vi "CL-close-CAN-test.vi"() -> ()   [LabVIEW 2016]
uses:
  <vilib>/Platform/TimedLoop/XDataNode/timing_clust.ctl
  <vilib>/Platform/TimedLoop/XDataNode/nitl_modes.ctl
  <vilib>/Platform/TimedLoop/XDataNode/wakeup.ctl
  <vilib>/xnet/xnet.llb/XNET Write (Signal Single-point).vi
  <vilib>/Platform/TimedLoop/XDataNode/XDataNode.xnode
  <vilib>/Platform/TimedLoop/XDataNode/XDNodeRunTimeDep.lvlib
panel:
  in  "Period":i64=10
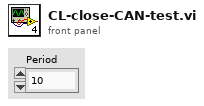
[diagram p1: front panel]
types:
  T1 = typedef "XDNodeRunTimeDep.lvlib/timing_clust.ctl" = cluster{"Expected End [f-1]":u64, "Actual End [f-1]":u64, "Finished Late? [f-1]":bool, "Expected End [i-1]":u64, "Actual End [i-1]":u64, "Finished Late? [i-1]":bool, "Expected Start [i]":u64, "Actual Start [i]":u64, "Expected Start [f]":u64, "Actual Start [f]":u64, "Source Name":string, "Structure Name":string, "Period":i64, "Deadline":i64, "Offset":i64, "Start":i64, "Priority":i32, "Timeout":i32, "Mode":T2, "Wakeup Reason":T3, "Error":errorcluster, "Source Type":string, "Secondary Source Type":string, "Global End Time":u64, "Global Start Time":u64, "Frame Duration":u64, "Iteration Duration":u64, "Assigned CPU":i32, "I/O Scan Engine Mode":u32}
  T2 = typedef "XDNodeRunTimeDep.lvlib/nitl_modes.ctl" = enum32{"No Change", "Process missed periods, maintain original phase", "Discard missed periods, maintain original phase", "Process missed periods, ignore original phase", "Discard missed periods, ignore original phase"}
  T3 = typedef "XDNodeRunTimeDep.lvlib/wakeup.ctl" = enum32{"Normal", "Aborted", "Asynchronous wakeup", "Timing source error", "Timed loop error", "Timeout"}
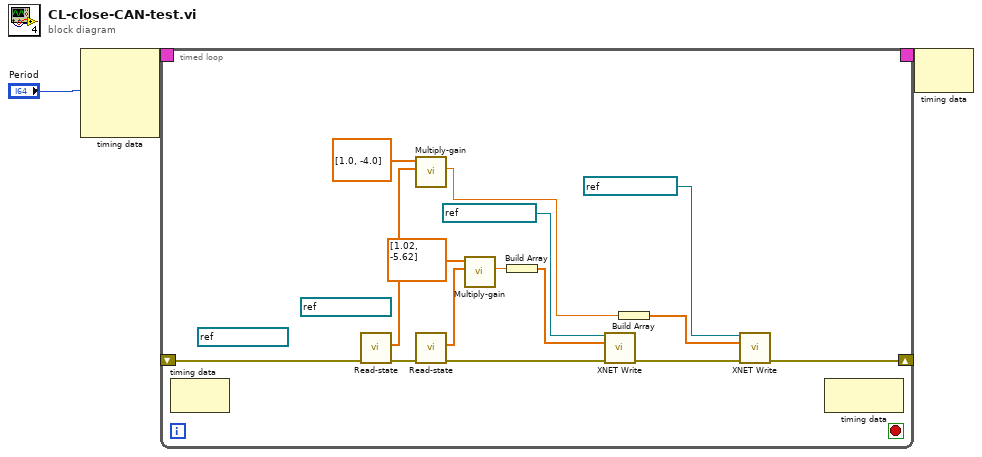
[diagram p0: block diagram]
diagram:
  n1 = node-c288("Period") -> (w3:T1)  [unwired: 3 in]
  n2 = timed-loop {
    timing: w3 -> [_]
    timing-out: [_] -> w2
    shift-right: [w10] -> _
    shift-left: _ -> [w17]
    stop <- _ stop-if-true
    (unwired) refnum<k21> "Plant2_state" ("XNET Session")
    (unwired) refnum<k21> "Plant1_state" ("XNET Session")
    n3 = node-c288() -> ()  [unwired: 1 in, 1 out]
    n4 = call "Read-state.vi"("error in (no error)"=w17) -> ("error out"=w18:errorcluster, "state"=w16:dbl[])  [unwired: 9 in]
    n5 = call "Multiply-gain.vi"("State (X)"=w16, "Gain (K)"=dbl[] [1.0, -4.0]) -> ("Kx"=w7:dbl)  [unwired: 9 in]
    n6 = call "Read-state.vi"("error in (no error)"=w18) -> ("error out"=w12:errorcluster, "state"=w13:dbl[])  [unwired: 9 in]
    n7 = call "Multiply-gain.vi"("State (X)"=w13, "Gain (K)"=dbl[] [1.02, -5.62]) -> ("Kx"=w6:dbl)  [unwired: 9 in]
    n8 = Build Array(w6) -> (w5:dbl[])
    n9 = call-poly <vilib>:"XNET Write.vi"("session in"=refnum<k21> "Plant2_Input", "data"=w5, "error in (no error)"=w12) -> ("error out"=w11:errorcluster)  [unwired: 11 in, 1 out]
    n10 = Build Array(w7) -> (w4:dbl[])
    n11 = call-poly <vilib>:"XNET Write.vi"("session in"=refnum<k21> "Plant1_Input", "data"=w4, "error in (no error)"=w11) -> ("error out"=w10:errorcluster)  [unwired: 11 in, 1 out]
    n12 = node-c288() -> ()  [unwired: 1 in, 1 out]
  }
  n13 = node-c288(w2) -> ()  [unwired: 1 out]
